vi "运维调试_五参数.vi"() -> ()   [LabVIEW 2016, in "斯坦道仪器.lvlib"]
uses:
  <vilib>/Utility/miscctls.llb/LVPointTypeDef.ctl
  PLC/PLC.lvlib
panel:
  in  "打开串口":bool
  in  "释放串口":bool
  in  "手动通电":bool
  out "多参数横条运行状态":T1(xcontrol)
  in  "数据区":i32(listbox)
  in  "探头选择":u16(ring)=9 items=["氨氮"=3, "水温"=9, "pH值"=10, "溶解氧"=11, "电导率"=12, "浊度"=13, "叶绿素a"=14, "藻密度"=15, "蓝绿藻"=16, "氧化还原电位"=17, "溶解氧%"=18, "盐度"=19]
  in  "测量数据区读取":bool
  in  "测量数据区":i32(listbox)
  in  "状态告警区读取":bool
  in  "状态告警区":i32(listbox)
  in  "自动校准":bool
  in  "读取KB":bool
  in  "写入KB":bool
  out "B":dbl caption="校准值B:"
  out "K":dbl caption="校准值K:"
  in  "校准区探头选择":u16(ring)=9 items=["氨氮"=3, "水温"=9, "pH值"=10, "电导率"=12, "浊度"=13, "叶绿素a"=14, "藻密度"=15, "蓝绿藻"=16, "氧化还原电位"=17, "溶解氧%"=18, "盐度"=19]
  in  "停止测量(单探)":bool
  in  "启动测量(单探)":bool
  in  "控制命令区探头选择":u16(ring)=9 items=["氨氮"=3, "水温"=9, "pH值"=10, "溶解氧"=11, "电导率"=12, "浊度"=13, "叶绿素a"=14, "藻密度"=15, "蓝绿藻"=16, "氧化还原电位"=17, "溶解氧%"=18, "盐度"=19]
  in  "同步时间":bool
  in  "初始化(清洗)":bool
  in  "停止测量(全部)":bool
  in  "启动测量(全部)":bool
  in  "关键参数区读取":bool
  in  "关键参数区":i32(listbox)
  in  "传感器参数读取":bool
  in  "传感器区":i32(listbox)
  in  "返回":bool
  in  "设置":bool
  out "运行状态":string
  out "开机状态":bool
  in  "停止":bool
  in  "手动启动":bool
  out "集成报警信息":string
  # "控制命令区"
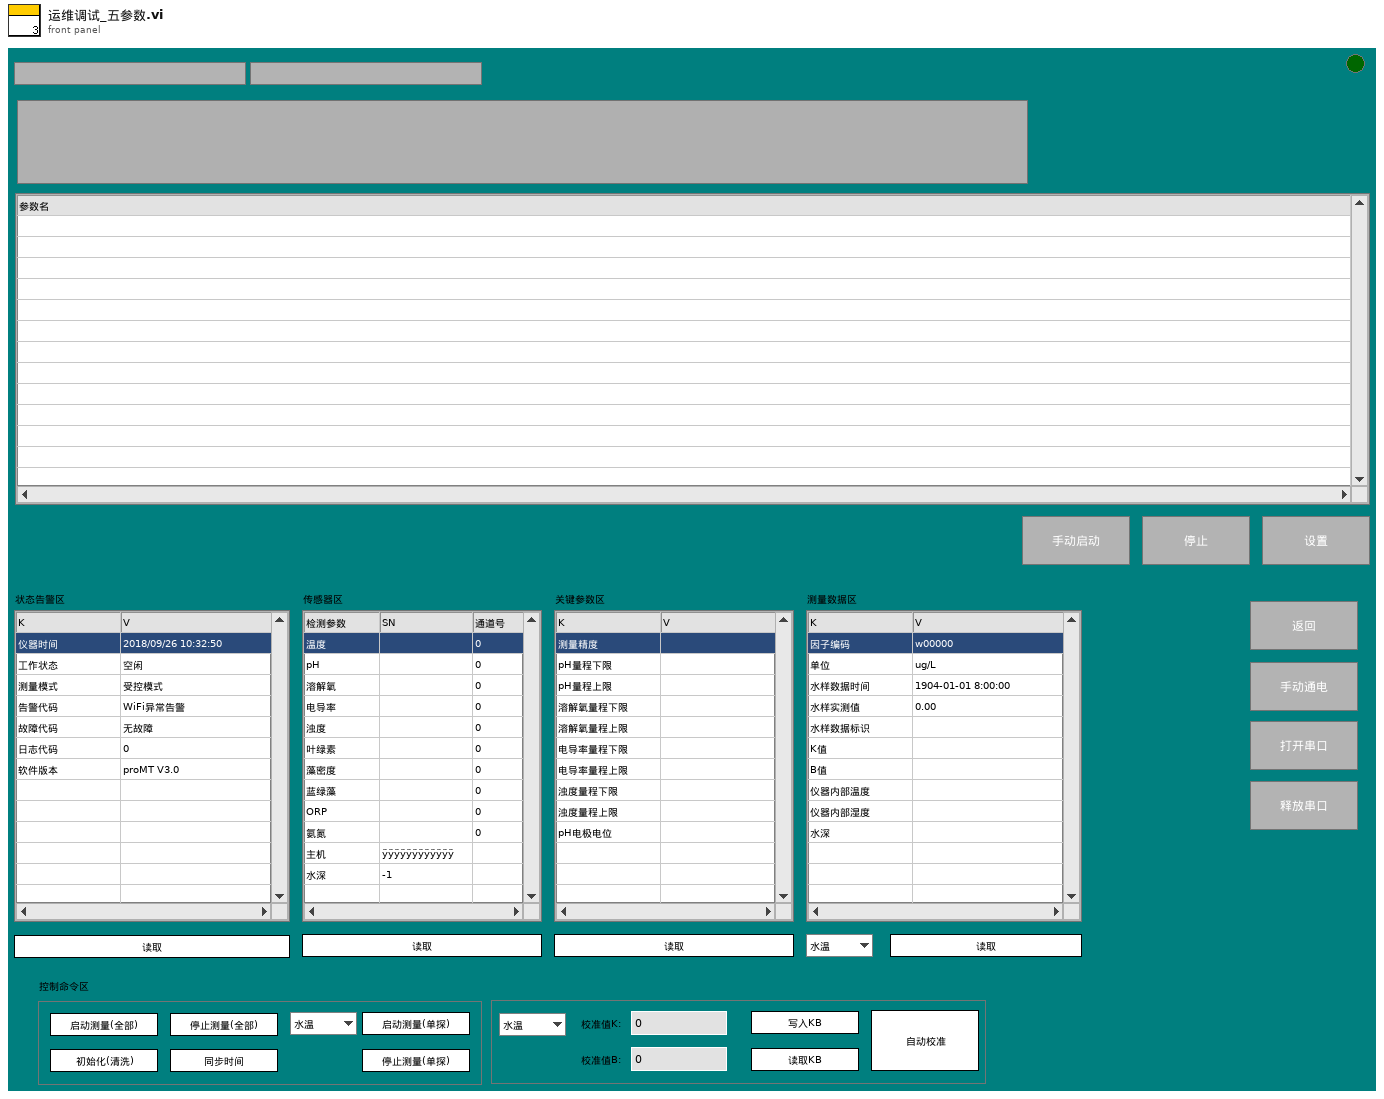
[diagram p1: front panel]
types:
  T1 = cluster{"系统时间":timestamp, "工作状态":u16, "测量模式":u16, "告警代码":enum16{"无告警", "缺试剂告警", "缺水样告警", "缺蒸馏水告警", "缺标液告警", "仪表漏液告警", "标定异常告警", "超量程告警", "加热异常", "低试剂预警", "超上限告警", "超下限告警", "仪表内部其他异常", "滴定异常告警", "电极异常告警", "量程切换告警", "参数设置告警", "PH电极电位异常", "电导率电极异常", "浊度光度异常", "溶解氧电极异常", "溶解氧光强异常", "温度异常告警", "PH异常告警", "溶解氧异常告警", "电导率异常告警", "浊度异常告警", "叶绿素异常告警", "藻密度异常告警", "蓝绿藻异常告警", "ORP异常告警", "氨氮异常告警", "清洁刷异常告警", "SD卡异常告警", "蓝牙异常告警", "Wifi异常告警", "流程异常告警"}, "故障代码":enum16{"无故障", "电机故障", "温度故障", "通讯故障", "滴定故障"}, "日志代码":u16, "软件版本":string}
  T2 = typedef "LVPointTypeDef.ctl" = cluster{"Horizontal":i16, "Vertical":i16}
  T3 = cluster{"时间标识":timestamp, "设备":string, "日志信息":string}
  T4 = enum16{"无告警", "缺试剂告警", "缺水样告警", "缺蒸馏水告警", "缺标液告警", "仪表漏液告警", "标定异常告警", "超量程告警", "加热异常", "低试剂预警", "超上限告警", "超下限告警", "仪表内部其他异常", "滴定异常告警", "电极异常告警", "量程切换告警", "参数设置告警", "PH电极电位异常", "电导率电极异常", "浊度光度异常", "溶解氧电极异常", "溶解氧光强异常", "温度异常告警", "PH异常告警", "溶解氧异常告警", "电导率异常告警", "浊度异常告警", "叶绿素异常告警", "藻密度异常告警", "蓝绿藻异常告警", "ORP异常告警", "氨氮异常告警", "清洁刷异常告警", "SD卡异常告警", "蓝牙异常告警", "Wifi异常告警", "流程异常告警"}
  T5 = cluster{"WORD[0]":u16, "WORD[1]":u16, "WORD[2]":u16, "WORD[3]":u16, "WORD[4]":u16, "WORD[5]":u16, "WORD[6]":u16, "WORD[7]":u16, "WORD[8]":u16, "WORD[9]":u16}
  T6 = cluster{"因子编码":string, "单位":string, "标样参考值":sgl, "水样数据时间":timestamp, "水样实测值":sgl, "水样数据标识":string, "K":sgl, "B":sgl, "T":sgl, "H":sgl, "水深":sgl}
  T7 = enum8{"Enabled", "Disabled", "Disabled and Grayed Out"}
  T8 = cluster{"测量模式":enum16{"待机", "水样测试", "标样核查", "零点核查", "跨度核查", "空白测试", "平行样测试", "加标回收", "空白校准", "标样校准", "初始化（清洗）"}, "数据标记表":string, "测量时间":dbl}
  T9 = cluster{"starting address":u16, "holding register value":u16}
  T10 = enum16{"idle", "init", "读状态", "读参数", "多个写入", "单个写入", "线圈写入"}
  T11 = enum32{"Bad", "Idle", "Run top level", "Running"}
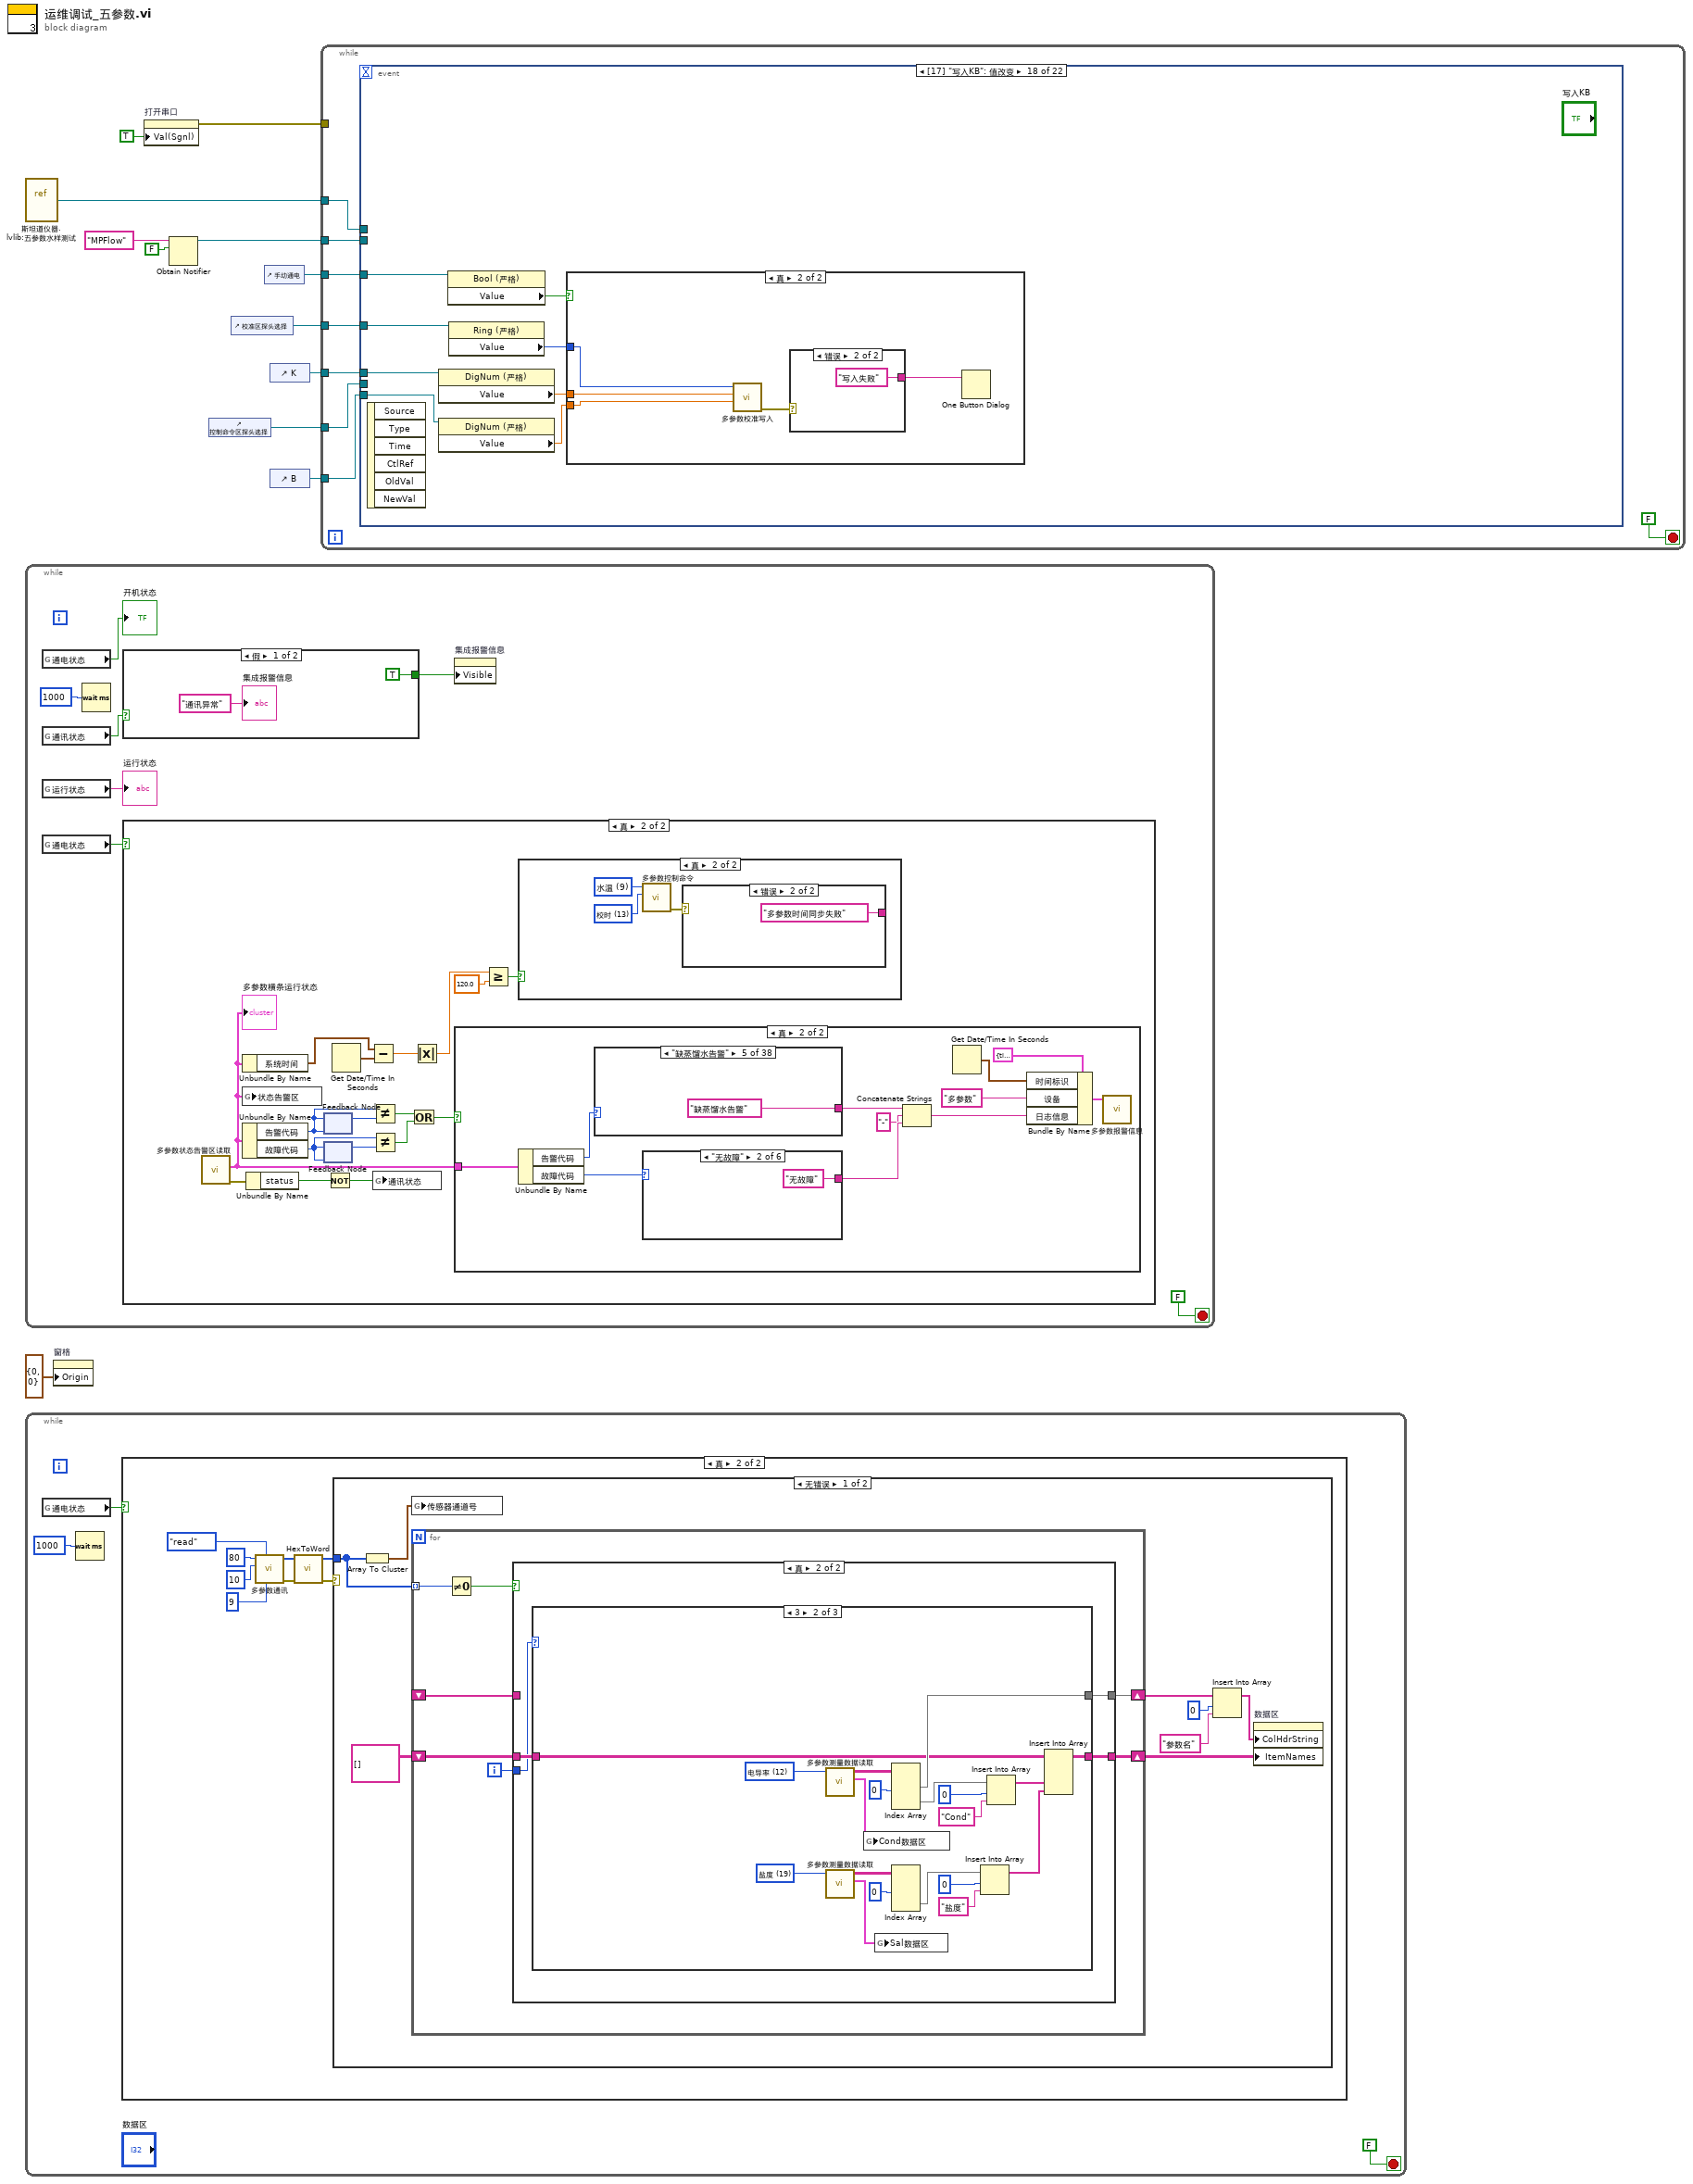
[diagram p0: block diagram]
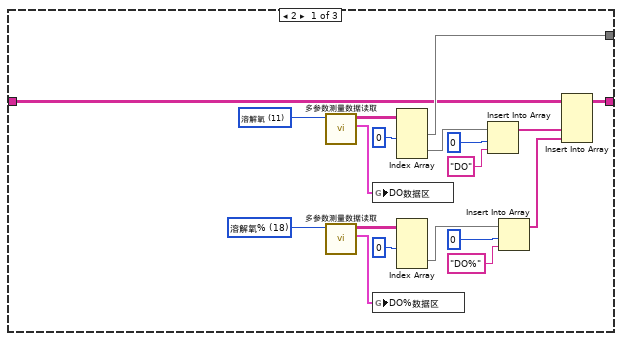
[diagram p4: hidden frame]
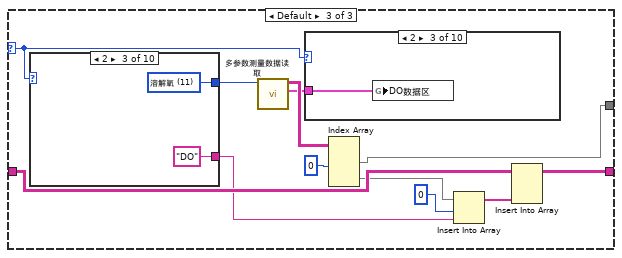
[diagram p5: hidden frame]
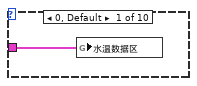
[diagram p6: hidden frame]
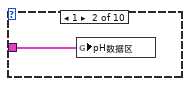
[diagram p7: hidden frame]
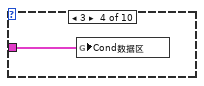
[diagram p8: hidden frame]
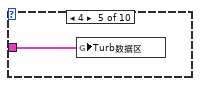
[diagram p9: hidden frame]
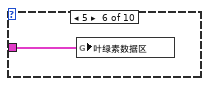
[diagram p10: hidden frame]
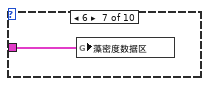
[diagram p11: hidden frame]
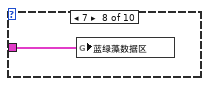
[diagram p12: hidden frame]
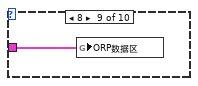
[diagram p13: hidden frame]
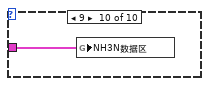
[diagram p14: hidden frame]
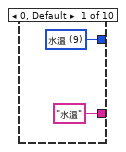
[diagram p15: hidden frame]
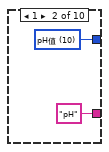
[diagram p16: hidden frame]
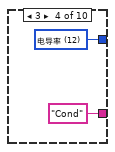
[diagram p17: hidden frame]
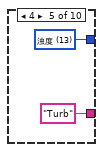
[diagram p18: hidden frame]
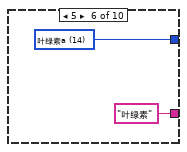
[diagram p19: hidden frame]
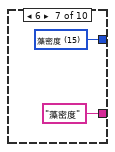
[diagram p20: hidden frame]
diagram:
  n1 = vi-ref "斯坦道仪器.lvlib:五参数水样测试.vi"() -> (w9:refnum<vi>)
  n2 = while {
    stop <- FALSE stop-if-true
    n3 = global read "多参数全局变量.vi" "通电状态"() -> (→"开机状态":bool)
    n4 = global read "多参数全局变量.vi" "通讯状态"() -> (w17:bool)
    n5 = global read "多参数全局变量.vi" "运行状态"() -> (→"运行状态":string)
    n6 = global read "多参数全局变量.vi" "通电状态"() -> (w13:bool)
    n7 = Wait (ms)(milliseconds to wait=u32 1000 ("等待时间（毫秒）")) -> ()  [unwired: 1 out]
    n8 = case shown="假" w17 {
      tunnel: [TRUE ("可见") _] -> w16
      frame False {
        "集成报警信息" <- "通讯异常" ("集成报警信息")
      }
      frame True {
      }
    }
    n9 = case shown="真" w13 {
      frame False {
      }
      frame True {
        n10 = call "多参数状态告警区读取.vi"() -> ("error out"=w29:errorcluster, "状态告警块"=w26:T1)  [unwired: 9 in, 1 out]
        "多参数横条运行状态" <- w26
        n11 = Unbundle By Name(w26) -> ("系统时间"=w25:timestamp)
        n12 = global write "多参数全局变量.vi" "状态告警区"(w26) -> ()
        n13 = Unbundle By Name(w26) -> ("告警代码"=w35:T4, "故障代码"=w33:enum16{"无故障", "电机故障", "温度故障", "通讯故障", "滴定故障"})
        n14 = Unbundle By Name(w29) -> ("status"=w28:bool)
        n15 = feedback #1(w35) -> (w36:T4)
        n16 = feedback-in #1(w35) -> ()
        n17 = feedback #2(w33) -> (w34:enum16{"无故障", "电机故障", "温度故障", "通讯故障", "滴定故障"})
        n18 = feedback-in #2(w33) -> ()
        n19 = Not(x=w28) -> (.not. x?=w27:bool)
        n20 = Get Date/Time In Seconds() -> (seconds since 1Jan1904=w24:timestamp)
        n21 = Subtract(x=w25, y=w24) -> (x-y=w23:dbl)
        n22 = Not Equal?(x=w35, y=w36) -> (x != y?=w31:bool)
        n23 = Not Equal?(x=w33, y=w34) -> (x != y?=w32:bool)
        n24 = global write "多参数全局变量.vi" "通讯状态"(w27) -> ()
        n25 = Or(x=w31, y=w32) -> (x .or. y?=w30:bool)
        n26 = Absolute Value(x=w23) -> (abs(x)=w22:dbl)
        n27 = case shown="真" w30 {
          tunnel: w26 -> [_ w52]
          frame False {
          }
          frame True {
            n28 = Unbundle By Name(w52) -> ("告警代码"=w51:T4, "故障代码"=w50:enum16{"无故障", "电机故障", "温度故障", "通讯故障", "滴定故障"})
            n29 = case shown="\"缺蒸馏水告警\"" w51 {
              selector: w51 -> [w63 _ _ _ _ _ _ _ _ _ _ _ _ _ _ _ _ _ _ _ _ _ _ _ _ _ _ _ _ _ _ _ _ _ _ _ _ _]
              tunnel: [w62 "无告警" "缺试剂告警" "缺水样告警" "缺蒸馏水告警" "缺标液告警" "仪表漏液告警" "标定异常告警" "超量程告警" "加热异常" "低试剂预警" "超上限告警" "超下限告警" "仪表内部其他异常" "滴定异常告警" "电极异常告警" "量程切换告警" "参数设置告警" "PH电极电位异常" "电导率电极异常" "浊度光度异常" "溶解氧电极异常" "溶解氧光强异常" "温度异常告警" "PH异常告警" "溶解氧异常告警" "电导率异常告警" "浊度异常告警" "叶绿素异常告警" "藻密度异常告警" "蓝绿藻异常告警" "ORP异常告警" "氨氮异常告警" "清洁刷异常告警" "SD卡异常告警" "蓝牙异常告警" "WiFi异常告警" "流程异常告警"] -> w49
              frame Default {
                n30 = Format Into String(format string="%d" ("格式字符串"), initial string="未知" ("工作状态"), w63) -> (resulting string=w62:string)  [unwired: 1 in, 1 out]
              }
              frame "无告警" {
              }
              frame "缺试剂告警" {
              }
              frame "缺水样告警" {
              }
              frame "缺蒸馏水告警" {
              }
              frame "缺标液告警" {
              }
              frame "仪表漏液告警" {
              }
              frame "标定异常告警" {
              }
              frame "超量程告警" {
              }
              frame "加热异常" {
              }
              frame "低试剂预警" {
              }
              frame "超上限告警" {
              }
              frame "超下限告警" {
              }
              frame "仪表内部其他异常" {
              }
              frame "滴定异常告警" {
              }
              frame "电极异常告警" {
              }
              frame "量程切换告警" {
              }
              frame "参数设置告警" {
              }
              frame "PH电极电位异常" {
              }
              frame "电导率电极异常" {
              }
              frame "浊度光度异常" {
              }
              frame "溶解氧电极异常" {
              }
              frame "溶解氧光强异常" {
              }
              frame "温度异常告警" {
              }
              frame "PH异常告警" {
              }
              frame "溶解氧异常告警" {
              }
              frame "电导率异常告警" {
              }
              frame "浊度异常告警" {
              }
              frame "叶绿素异常告警" {
              }
              frame "藻密度异常告警" {
              }
              frame "蓝绿藻异常告警" {
              }
              frame "ORP异常告警" {
              }
              frame "氨氮异常告警" {
              }
              frame "清洁刷异常告警" {
              }
              frame "SD卡异常告警" {
              }
              frame "蓝牙异常告警" {
              }
              frame "Wifi异常告警" {
              }
              frame "流程异常告警" {
              }
            }
            n31 = case shown="\"无故障\"" w50 {
              selector: w50 -> [w54 _ _ _ _ _]
              tunnel: [w53 "无故障" "电机故障" "温度故障" "通讯故障" "滴定故障"] -> w48
              frame Default {
                n32 = Format Into String(format string="%d" ("格式字符串"), initial string="未知" ("工作状态"), w54) -> (resulting string=w53:string)  [unwired: 1 in, 1 out]
              }
              frame "无故障" {
              }
              frame "电机故障" {
              }
              frame "温度故障" {
              }
              frame "通讯故障" {
              }
              frame "滴定故障" {
              }
            }
            n33 = Concatenate Strings(w49, "-" ("字符串"), w48) -> (w44:string)
            n34 = Get Date/Time In Seconds() -> (seconds since 1Jan1904=w43:timestamp)
            n35 = Bundle By Name(cluster=T3 {"时间标识"=timestamp(0 s since 1904-01-01), "设备"="", "日志信息"=""} ("data in"), "时间标识"=w43, "设备"="多参数", "日志信息"=w44) -> (w45:T3)
            n36 = call "多参数报警信息.vi"("data in"=w45) -> ()  [unwired: 10 in, 1 out]
          }
        }
        n37 = Greater Or Equal?(x=w22, y=120.0) -> (x >= y?=w21:bool)
        n38 = case shown="真" w21 {
          frame False {
          }
          frame True {
            w37 = u16 13 items=["启动测量（全部）"=1, "初始化（清洗）"=10, "停止测量（全部）"=11, "校时"=13, "启动测量（单个传感器）"=19, "停止测量（单个传感器）"=20] ("控制命令")
            w38 = u16 9 items=["氨氮"=3, "水温"=9, "pH值"=10, "溶解氧"=11, "电导率"=12, "浊度"=13, "叶绿素a"=14, "藻密度"=15, "蓝绿藻"=16, "氧化还原电位"=17, "溶解氧%"=18, "盐度"=19] ("站号")
            n39 = call "多参数控制命令.vi"("控制命令"=w37, "站号"=w38) -> ("error out"=w39:errorcluster)  [unwired: 9 in]
            n40 = case shown="错误" w39 {
              tunnel: ["多参数时间同步成功" ("消息") "多参数时间同步失败" ("消息")] -> _
              frame No Error {
              }
              frame Error {
              }
            }
          }
        }
      }
    }
    n41 = property on="集成报警信息" class="Str"("Visible"=w16) -> ()  [unwired: 2 in, 2 out]
  }
  n42 = while {
    stop <- FALSE stop-if-true
    n43 = global read "多参数全局变量.vi" "通电状态"() -> (w105:bool)
    n44 = Wait (ms)(milliseconds to wait=u32 1000 ("等待时间（毫秒）")) -> ()  [unwired: 1 out]
    n45 = case shown="真" w105 {
      frame False {
      }
      frame True {
        n46 = call "多参数通讯.vi"("Slave ID"=u8 9, "STEP"=enum16{"open", "read", "write", "close"}."read", "quantity"=u16 10, "starting address"=u16 80) -> ("error out"=w110:errorcluster, "Registers"=w111:u16[])  [unwired: 5 in, 1 out]
        n47 = call "HexToWord.vi"("数组"=w111) -> ("WORD"=w114:u16[])  [unwired: 10 in]
        n48 = case shown="无错误" w110 {
          tunnel: w114 -> [w115 _]
          frame No Error {
            n49 = Array To Cluster(array=w115) -> (cluster=w116:T5)
            n50 = global write "多参数全局变量.vi" "传感器通道号"(w116) -> ()
            n51 = for {
              tunnel: w115 -> [w128] mode=indexing
              shift-right: [w126] -> w120
              shift-left: _ -> [w125]
              shift-right: [w123] -> w121
              shift-left: string[][] [] ("子数组") -> [w124]
              i -> [w129]
              n52 = Not Equal To 0?(x=w128) -> (x != 0?=w127:bool)
              n53 = case shown="真" w127 {
                tunnel: w129 -> [_ w132]
                tunnel: [w131 w135] -> w126
                tunnel: w125 -> [w131 _]
                tunnel: w124 -> [w130 w134]
                tunnel: [w130 w133] -> w123
                frame False {
                }
                frame True {
                  n54 = case shown="3" w132 {
                    selector: w132 -> [_ _ w174]
                    tunnel: [w144 w163 w182] -> w135
                    tunnel: w134 -> [w140 w159 w181]
                    tunnel: [w143 w162 w180] -> w133
                    frame 2 {
                      w138 = u16 18 items=["氨氮"=3, "水温"=9, "pH值"=10, "溶解氧"=11, "电导率"=12, "浊度"=13, "叶绿素a"=14, "藻密度"=15, "蓝绿藻"=16, "氧化还原电位"=17, "溶解氧%"=18, "盐度"=19] ("探头选择")
                      w139 = u16 11 items=["氨氮"=3, "水温"=9, "pH值"=10, "溶解氧"=11, "电导率"=12, "浊度"=13, "叶绿素a"=14, "藻密度"=15, "蓝绿藻"=16, "氧化还原电位"=17, "溶解氧%"=18, "盐度"=19] ("探头选择")
                      n55 = call "多参数测量数据读取.vi"("探头选择"=w139) -> ("测量数据块"=w137:T6, "添加的数组"=w142:string[][])  [unwired: 8 in, 1 out]
                      n56 = call "多参数测量数据读取.vi"("探头选择"=w138) -> ("测量数据块"=w136:T6, "添加的数组"=w141:string[][])  [unwired: 8 in, 1 out]
                      n57 = global write "多参数全局变量.vi" "DO数据区"(w137) -> ()
                      n58 = global write "多参数全局变量.vi" "DO%数据区"(w136) -> ()
                      n59 = Index Array(array=w142, index (col) #1=0 ("禁用的索引 (列)")) -> (element #1=w144:string[], element #2=w153:string[])  [unwired: 3 in]
                      n60 = Index Array(array=w141, index (col) #1=0 ("禁用的索引 (列)")) -> (element #2=w149:string[])  [unwired: 3 in, 1 out]
                      n61 = Insert Into Array(array=w153, index=0 ("索引"), new element="DO") -> (w151:string[])
                      n62 = Insert Into Array(array=w149, index=0 ("索引"), new element="DO%") -> (w148:string[])
                      n63 = Insert Into Array(array=w140, new element #1=w151, new element #2=w148) -> (w143:string[][])  [unwired: 2 in]
                    }
                    frame 3 {
                      w157 = u16 19 items=["氨氮"=3, "水温"=9, "pH值"=10, "溶解氧"=11, "电导率"=12, "浊度"=13, "叶绿素a"=14, "藻密度"=15, "蓝绿藻"=16, "氧化还原电位"=17, "溶解氧%"=18, "盐度"=19] ("探头选择")
                      w158 = u16 12 items=["氨氮"=3, "水温"=9, "pH值"=10, "溶解氧"=11, "电导率"=12, "浊度"=13, "叶绿素a"=14, "藻密度"=15, "蓝绿藻"=16, "氧化还原电位"=17, "溶解氧%"=18, "盐度"=19] ("探头选择")
                      n64 = call "多参数测量数据读取.vi"("探头选择"=w158) -> ("测量数据块"=w156:T6, "添加的数组"=w161:string[][])  [unwired: 8 in, 1 out]
                      n65 = call "多参数测量数据读取.vi"("探头选择"=w157) -> ("测量数据块"=w155:T6, "添加的数组"=w160:string[][])  [unwired: 8 in, 1 out]
                      n66 = global write "多参数全局变量.vi" "Cond数据区"(w156) -> ()
                      n67 = global write "多参数全局变量.vi" "Sal数据区"(w155) -> ()
                      n68 = Index Array(array=w161, index (col) #1=0 ("禁用的索引 (列)")) -> (element #1=w163:string[], element #2=w172:string[])  [unwired: 3 in]
                      n69 = Index Array(array=w160, index (col) #1=0 ("禁用的索引 (列)")) -> (element #2=w168:string[])  [unwired: 3 in, 1 out]
                      n70 = Insert Into Array(array=w168, index=0 ("索引"), new element="盐度") -> (w167:string[])
                      n71 = Insert Into Array(array=w172, index=0 ("索引"), new element="Cond") -> (w170:string[])
                      n72 = Insert Into Array(array=w159, new element #1=w170, new element #2=w167) -> (w162:string[][])  [unwired: 2 in]
                    }
                    frame Default {
                      n73 = case shown="2" w174 {
                        tunnel: [w197 w199 w201 w203 w205 w207 w209 w211 w213 w215] -> w185
                        tunnel: ["水温" "pH" "DO" "Cond" "Turb" "叶绿素" "藻密度" "蓝绿藻" "ORP" "氨氮"] -> w178
                        frame 0, Default {
                          w197 = u16 9 items=["氨氮"=3, "水温"=9, "pH值"=10, "溶解氧"=11, "电导率"=12, "浊度"=13, "叶绿素a"=14, "藻密度"=15, "蓝绿藻"=16, "氧化还原电位"=17, "溶解氧%"=18, "盐度"=19] ("探头选择")
                        }
                        frame 1 {
                          w199 = u16 10 items=["氨氮"=3, "水温"=9, "pH值"=10, "溶解氧"=11, "电导率"=12, "浊度"=13, "叶绿素a"=14, "藻密度"=15, "蓝绿藻"=16, "氧化还原电位"=17, "溶解氧%"=18, "盐度"=19] ("探头选择")
                        }
                        frame 2 {
                          w201 = u16 11 items=["氨氮"=3, "水温"=9, "pH值"=10, "溶解氧"=11, "电导率"=12, "浊度"=13, "叶绿素a"=14, "藻密度"=15, "蓝绿藻"=16, "氧化还原电位"=17, "溶解氧%"=18, "盐度"=19] ("探头选择")
                        }
                        frame 3 {
                          w203 = u16 12 items=["氨氮"=3, "水温"=9, "pH值"=10, "溶解氧"=11, "电导率"=12, "浊度"=13, "叶绿素a"=14, "藻密度"=15, "蓝绿藻"=16, "氧化还原电位"=17, "溶解氧%"=18, "盐度"=19] ("探头选择")
                        }
                        frame 4 {
                          w205 = u16 13 items=["氨氮"=3, "水温"=9, "pH值"=10, "溶解氧"=11, "电导率"=12, "浊度"=13, "叶绿素a"=14, "藻密度"=15, "蓝绿藻"=16, "氧化还原电位"=17, "溶解氧%"=18, "盐度"=19] ("探头选择")
                        }
                        frame 5 {
                          w207 = u16 14 items=["氨氮"=3, "水温"=9, "pH值"=10, "溶解氧"=11, "电导率"=12, "浊度"=13, "叶绿素a"=14, "藻密度"=15, "蓝绿藻"=16, "氧化还原电位"=17, "溶解氧%"=18, "盐度"=19] ("探头选择")
                        }
                        frame 6 {
                          w209 = u16 15 items=["氨氮"=3, "水温"=9, "pH值"=10, "溶解氧"=11, "电导率"=12, "浊度"=13, "叶绿素a"=14, "藻密度"=15, "蓝绿藻"=16, "氧化还原电位"=17, "溶解氧%"=18, "盐度"=19] ("探头选择")
                        }
                        frame 7 {
                          w211 = u16 16 items=["氨氮"=3, "水温"=9, "pH值"=10, "溶解氧"=11, "电导率"=12, "浊度"=13, "叶绿素a"=14, "藻密度"=15, "蓝绿藻"=16, "氧化还原电位"=17, "溶解氧%"=18, "盐度"=19] ("探头选择")
                        }
                        frame 8 {
                          w213 = u16 17 items=["氨氮"=3, "水温"=9, "pH值"=10, "溶解氧"=11, "电导率"=12, "浊度"=13, "叶绿素a"=14, "藻密度"=15, "蓝绿藻"=16, "氧化还原电位"=17, "溶解氧%"=18, "盐度"=19] ("探头选择")
                        }
                        frame 9 {
                          w215 = u16 3 items=["氨氮"=3, "水温"=9, "pH值"=10, "溶解氧"=11, "电导率"=12, "浊度"=13, "叶绿素a"=14, "藻密度"=15, "蓝绿藻"=16, "氧化还原电位"=17, "溶解氧%"=18, "盐度"=19] ("探头选择")
                        }
                      }
                      n74 = call "多参数测量数据读取.vi"("探头选择"=w185) -> ("测量数据块"=w175:T6, "添加的数组"=w184:string[][])  [unwired: 8 in, 1 out]
                      n75 = case shown="2" w174 {
                        tunnel: w175 -> [w186 w187 w188 w189 w190 w191 w192 w193 w194 w195]
                        frame 0, Default {
                          n76 = global write "多参数全局变量.vi" "水温数据区"(w186) -> ()
                        }
                        frame 1 {
                          n77 = global write "多参数全局变量.vi" "pH数据区"(w187) -> ()
                        }
                        frame 2 {
                          n78 = global write "多参数全局变量.vi" "DO数据区"(w188) -> ()
                        }
                        frame 3 {
                          n79 = global write "多参数全局变量.vi" "Cond数据区"(w189) -> ()
                        }
                        frame 4 {
                          n80 = global write "多参数全局变量.vi" "Turb数据区"(w190) -> ()
                        }
                        frame 5 {
                          n81 = global write "多参数全局变量.vi" "叶绿素数据区"(w191) -> ()
                        }
                        frame 6 {
                          n82 = global write "多参数全局变量.vi" "藻密度数据区"(w192) -> ()
                        }
                        frame 7 {
                          n83 = global write "多参数全局变量.vi" "蓝绿藻数据区"(w193) -> ()
                        }
                        frame 8 {
                          n84 = global write "多参数全局变量.vi" "ORP数据区"(w194) -> ()
                        }
                        frame 9 {
                          n85 = global write "多参数全局变量.vi" "NH3N数据区"(w195) -> ()
                        }
                      }
                      n86 = Index Array(array=w184, index (col) #1=0 ("禁用的索引 (列)")) -> (element #1=w182:string[], element #2=w179:string[])  [unwired: 3 in]
                      n87 = Insert Into Array(array=w179, index=0 ("索引"), new element=w178) -> (w177:string[])
                      n88 = Insert Into Array(array=w181, new element=w177) -> (w180:string[][])  [unwired: 2 in]
                    }
                  }
                }
              }
            }
            n89 = Insert Into Array(array=w120, index=0 ("索引"), new element="参数名" ("新元素/子数组")) -> (w119:string[])
            n90 = property on="数据区" class="MCListbox (严格)"("ColHdrString"=w119, "ItemNames"=w121) -> ()  [unwired: 2 in, 2 out]
          }
          frame Error {
          }
        }
      }
    }
  }
  n91 = property on="窗格" class="Pane"("Origin"=T2 {"Horizontal"=0, "Vertical"=0} ("原点")) -> ()  [unwired: 2 in, 2 out]
  n92 = property on="打开串口" class="Bool (严格)"("Val(Sgnl)"=TRUE ("值(信号)")) -> (error out=w1:errorcluster)  [unwired: 2 in, 1 out]
  n93 = Obtain Notifier(name (unnamed)="MPFlow" ("名称（未命名）"), notification data type=FALSE) -> (notifier out=w8:refnum<notifier>)  [unwired: 2 in, 2 out]
  n94 = control-ref of="控制命令区探头选择"() -> (w7:refnum<vi>)
  n95 = control-ref of="校准区探头选择"() -> (w4:refnum<vi>)
  n96 = control-ref of="手动通电"() -> (w3:refnum<vi>)
  n97 = control-ref of="K"() -> (w6:refnum<vi>)
  n98 = control-ref of="B"() -> (w5:refnum<vi>)
  n99 = while {
    tunnel: w9 -> [w222]
    tunnel: w8 -> [w221]
    tunnel: w7 -> [w220]
    tunnel: w6 -> [w219]
    tunnel: w5 -> [w218]
    tunnel: w4 -> [w217]
    tunnel: w3 -> [w216]
    tunnel: w1 -> [_]
    stop <- FALSE stop-if-true
    n100 = event shown="[17] \"写入KB\": 值改变" {
      selector: _ -> [_ _ _ _ _ _ _ _ _ _ _ _ _ _ _ _ _ _ _ _ _ _]
      dyn-events: _ -> [_ _ _ _ _ _ _ _ _ _ _ _ _ _ _ _ _ _ _ _ _ _]
      timeout: _ -> [_ _ _ _ _ _ _ _ _ _ _ _ _ _ _ _ _ _ _ _ _ _]
      tunnel: w222 -> [_ _ _ w238 _ _ _ _ _ _ _ _ _ _ _ _ _ _ _ _ _ _]
      tunnel: w221 -> [_ _ _ _ w260 _ _ _ _ _ _ _ _ _ _ _ _ _ _ _ _ _]
      tunnel: w220 -> [_ _ _ _ _ _ _ _ _ _ _ _ _ _ _ w324 w338 _ _ _ _ _]
      tunnel: w219 -> [_ _ _ _ _ _ _ _ _ _ _ _ _ _ _ _ _ w349 _ _ _ _]
      tunnel: w218 -> [_ _ _ _ _ _ _ _ _ _ _ _ _ _ _ _ _ w351 _ _ _ _]
      tunnel: w217 -> [_ _ _ _ _ _ _ _ _ _ _ _ _ _ _ _ _ w353 _ w369 _ _]
      tunnel: w216 -> [_ _ _ _ _ _ _ w268 w273 w278 w284 w289 w298 w307 w316 w326 w336 w347 _ w367 w379 _]
      event Timeout {
        n101 = event-data() -> ()  [unwired: 1 in, 3 out]
      }
      event "释放串口": Value Change {
        n102 = event-data() -> ("NewVal"=w224:bool)  [unwired: 1 in, 5 out]
        n103 = case shown="真" w224 {
          frame False {
          }
          frame True {
            n104 = call "多参数通讯.vi"("STEP"=enum16{"open", "read", "write", "close"}."close") -> ("error out"=w225:errorcluster)  [unwired: 8 in, 2 out]
            n105 = case shown="无错误" w225 {
              frame No Error {
                n106 = property on="打开串口" class="Bool (严格)"("DisabledEnum"=T7."Enabled" ("禁用")) -> ()  [unwired: 2 in, 2 out]
              }
              frame Error {
              }
            }
          }
        }
      }
      event "打开串口": Value Change {
        n107 = event-data() -> ("NewVal"=w228:bool)  [unwired: 1 in, 5 out]
        n108 = case shown="真" w228 {
          frame False {
          }
          frame True {
            n109 = call "多参数通讯.vi"("STEP"=enum16{"open", "read", "write", "close"}."open") -> ("error out"=w229:errorcluster)  [unwired: 8 in, 2 out]
            n110 = case shown="错误" w229 {
              tunnel: [T7."Disabled and Grayed Out" ("禁用") T7."Enabled" ("禁用")] -> w231
              frame No Error {
              }
              frame Error {
                n111 = One Button Dialog(message="多参数串口打开失败" ("消息")) -> ()  [unwired: 1 in, 1 out]
              }
            }
            n112 = property on="打开串口" class="Bool (严格)"("DisabledEnum"=w231, "Value"=FALSE ("打开串口")) -> ()  [unwired: 2 in, 2 out]
          }
        }
      }
      event "手动启动": Value Change {
        n113 = event-data() -> ()  [unwired: 1 in, 6 out]
        n114 = call "多参数启动参数对话框.vi"() -> ("确认"=w237:bool, "测量时间"=w236:dbl)  [unwired: 10 in]
        n115 = case shown="真" w237 {
          tunnel: w238 -> [_ w240]
          tunnel: w236 -> [_ w239]
          frame False {
          }
          frame True {
            n116 = property class="VI"(reference=w240) -> ("Name"=w244:string, "Exec.State"=w242:T11)  [unwired: 1 in, 2 out]
            n117 = Open VI Reference(type specifier VI Refnum (for type only)=refnum<vi> refnum ("类型说明符VI引用句柄（仅用于类型）"), vi path=w244, options=128 ("选项")) -> (vi reference=w243:refnum<vi>)  [unwired: 3 in, 1 out]
            n118 = case shown="\"Idle\"" w242 {
              tunnel: w243 -> [w248 w255]
              tunnel: [w248 w254] -> w241
              tunnel: w239 -> [_ w249]
              frame "Bad", Default {
                n119 = One Button Dialog(message="仪器已经启动，无需重复启动" ("消息")) -> ()  [unwired: 1 in, 1 out]
              }
              frame "Idle" {
                n120 = global read "系统变量.vi" "运行模式"() -> (w251:enum16{"维护模式", "常规模式", "应急模式", "质控模式"})
                n121 = case shown="\"常规模式\", 默认" w251 {
                  tunnel: ["M" ("数据标记表") "hd" ("数据标记表")] -> w250
                  frame "维护模式" {
                  }
                  frame "常规模式", Default {
                  }
                }
                n122 = Bundle By Name(cluster=T8 {"测量模式"=enum."水样测试", "数据标记表"="", "测量时间"=0.0} ("启动参数"), "数据标记表"=w250, "测量时间"=w249) -> (w252:T8)
                n123 = call-by-ref "开始异步调用"(reference=w255, "启动参数"=w252) -> (reference out=w254:refnum<vi>)  [unwired: 12 in, 1 out]
              }
            }
            n124 = Close Reference(reference=w241) -> ()  [unwired: 1 in, 1 out]
          }
        }
      }
      event "停止": Value Change {
        n125 = event-data() -> ()  [unwired: 1 in, 6 out]
        n126 = Two Button Dialog(message="请再一次确认是否停止测量" ("消息")) -> (T button?=w258:bool)  [unwired: 2 in]
        n127 = case shown="真" w258 {
          tunnel: w260 -> [_ w263]
          frame False {
          }
          frame True {
            w261 = u16 11 items=["启动测量（全部）"=1, "初始化（清洗）"=10, "停止测量（全部）"=11, "校时"=13, "启动测量（单个传感器）"=19, "停止测量（单个传感器）"=20] ("控制命令")
            w262 = u16 10 items=["氨氮"=3, "水温"=9, "pH值"=10, "溶解氧"=11, "电导率"=12, "浊度"=13, "叶绿素a"=14, "藻密度"=15, "蓝绿藻"=16, "氧化还原电位"=17, "溶解氧%"=18, "盐度"=19] ("站号")
            n128 = Send Notification(notification=TRUE ("通知"), notifier=w263) -> ()  [unwired: 1 in, 2 out]
            n129 = call "多参数控制命令.vi"("控制命令"=w261, "站号"=w262) -> ()  [unwired: 9 in, 1 out]
          }
        }
      }
      event "设置": Value Change {
        n130 = event-data() -> ()  [unwired: 1 in, 6 out]
        n131 = property on="窗格" class="Pane"("Origin"=T2 {"Horizontal"=0, "Vertical"=528} ("原点")) -> ()  [unwired: 2 in, 2 out]
      }
      event "返回": Value Change {
        n132 = event-data() -> ()  [unwired: 1 in, 6 out]
        n133 = property on="窗格" class="Pane"("Origin"=T2 {"Horizontal"=0, "Vertical"=0} ("原点")) -> ()  [unwired: 2 in, 2 out]
      }
      event "传感器参数读取": Value Change {
        n134 = event-data() -> ()  [unwired: 1 in, 6 out]
        n135 = property class="Bool (严格)"(reference=w268) -> ("Value"=w267:bool)  [unwired: 1 in, 2 out]
        n136 = case shown="真" w267 {
          frame False {
            n137 = One Button Dialog(message="启动失败，请先通电" ("消息")) -> ()  [unwired: 1 in, 1 out]
          }
          frame True {
            n138 = call "多参数传感器参数读取.vi"() -> ("error out"=w270:errorcluster, "添加的数组"=w271:string[][])  [unwired: 10 in]
            n139 = call <vilib>:"General Error Handler.vi"("error in (no error)"=w270) -> ()  [unwired: 10 in, 5 out]
            n140 = property on="传感器区" class="MCListbox (严格)"("ItemNames"=w271) -> ()  [unwired: 2 in, 2 out]
          }
        }
      }
      event "关键参数区读取": Value Change {
        n141 = event-data() -> ()  [unwired: 1 in, 6 out]
        n142 = property class="Bool (严格)"(reference=w273) -> ("Value"=w272:bool)  [unwired: 1 in, 2 out]
        n143 = case shown="假" w272 {
          frame False {
            n144 = One Button Dialog(message="启动失败，请先通电" ("消息")) -> ()  [unwired: 1 in, 1 out]
          }
          frame True {
            n145 = call "多参数关键参数读取.vi"() -> ("error out"=w275:errorcluster, "添加的数组"=w276:string[][])  [unwired: 10 in]
            n146 = call <vilib>:"General Error Handler.vi"("error in (no error)"=w275) -> ()  [unwired: 10 in, 5 out]
            n147 = property on="关键参数区" class="MCListbox (严格)"("ItemNames"=w276) -> ()  [unwired: 2 in, 2 out]
          }
        }
      }
      event "测量数据区读取": Value Change {
        n148 = event-data() -> ()  [unwired: 1 in, 6 out]
        n149 = property class="Bool (严格)"(reference=w278) -> ("Value"=w277:bool)  [unwired: 1 in, 2 out]
        n150 = case shown="假" w277 {
          frame False {
            n151 = One Button Dialog(message="启动失败，请先通电" ("消息")) -> ()  [unwired: 1 in, 1 out]
          }
          frame True {
            n152 = call "多参数测量数据读取.vi"("探头选择"="探头选择") -> ("error out"=w281:errorcluster, "添加的数组"=w282:string[][])  [unwired: 8 in, 1 out]
            n153 = call <vilib>:"General Error Handler.vi"("error in (no error)"=w281) -> ()  [unwired: 10 in, 5 out]
            n154 = property on="测量数据区" class="MCListbox (严格)"("ItemNames"=w282) -> ()  [unwired: 2 in, 2 out]
          }
        }
      }
      event "状态告警区读取": Value Change {
        n155 = event-data() -> ()  [unwired: 1 in, 6 out]
        n156 = property class="Bool (严格)"(reference=w284) -> ("Value"=w283:bool)  [unwired: 1 in, 2 out]
        n157 = case shown="真" w283 {
          frame False {
            n158 = One Button Dialog(message="启动失败，请先通电" ("消息")) -> ()  [unwired: 1 in, 1 out]
          }
          frame True {
            n159 = call "多参数状态告警区读取.vi"() -> ("error out"=w286:errorcluster, "添加的数组"=w287:string[][])  [unwired: 9 in, 1 out]
            n160 = call <vilib>:"General Error Handler.vi"("error in (no error)"=w286) -> ()  [unwired: 10 in, 5 out]
            n161 = property on="状态告警区" class="MCListbox (严格)"("ItemNames"=w287) -> ()  [unwired: 2 in, 2 out]
          }
        }
      }
      event "同步时间": Value Change {
        n162 = event-data() -> ()  [unwired: 1 in, 6 out]
        n163 = property class="Bool (严格)"(reference=w289) -> ("Value"=w288:bool)  [unwired: 1 in, 2 out]
        n164 = case shown="假" w288 {
          frame False {
            n165 = One Button Dialog(message="启动失败，请先通电" ("消息")) -> ()  [unwired: 1 in, 1 out]
          }
          frame True {
            w291 = u16 13 items=["启动测量（全部）"=1, "初始化（清洗）"=10, "停止测量（全部）"=11, "校时"=13, "启动测量（单个传感器）"=19, "停止测量（单个传感器）"=20] ("控制命令")
            w292 = u16 9 items=["氨氮"=3, "水温"=9, "pH值"=10, "溶解氧"=11, "电导率"=12, "浊度"=13, "叶绿素a"=14, "藻密度"=15, "蓝绿藻"=16, "氧化还原电位"=17, "溶解氧%"=18, "盐度"=19] ("站号")
            n166 = call "多参数控制命令.vi"("控制命令"=w291, "站号"=w292) -> ("error out"=w294:errorcluster)  [unwired: 9 in]
            n167 = case shown="错误" w294 {
              tunnel: ["时间同步成功" ("消息") "时间同步失败" ("消息")] -> w293
              frame No Error {
              }
              frame Error {
              }
            }
            n168 = One Button Dialog(message=w293) -> ()  [unwired: 1 in, 1 out]
          }
        }
      }
      event "启动测量(全部)": Value Change {
        n169 = event-data() -> ()  [unwired: 1 in, 6 out]
        n170 = property class="Bool (严格)"(reference=w298) -> ("Value"=w297:bool)  [unwired: 1 in, 2 out]
        n171 = case shown="假" w297 {
          frame False {
            n172 = One Button Dialog(message="启动失败，请先通电" ("消息")) -> ()  [unwired: 1 in, 1 out]
          }
          frame True {
            w300 = u16 1 items=["启动测量（全部）"=1, "初始化（清洗）"=10, "停止测量（全部）"=11, "校时"=13, "启动测量（单个传感器）"=19, "停止测量（单个传感器）"=20] ("控制命令")
            w301 = u16 9 items=["氨氮"=3, "水温"=9, "pH值"=10, "溶解氧"=11, "电导率"=12, "浊度"=13, "叶绿素a"=14, "藻密度"=15, "蓝绿藻"=16, "氧化还原电位"=17, "溶解氧%"=18, "盐度"=19] ("站号")
            n173 = call "多参数控制命令.vi"("控制命令"=w300, "站号"=w301) -> ("error out"=w303:errorcluster)  [unwired: 9 in]
            n174 = case shown="无错误" w303 {
              tunnel: ["启动成功" ("消息") "启动失败" ("消息")] -> w302
              frame No Error {
              }
              frame Error {
              }
            }
            n175 = One Button Dialog(message=w302) -> ()  [unwired: 1 in, 1 out]
          }
        }
      }
      event "停止测量(全部)": Value Change {
        n176 = event-data() -> ()  [unwired: 1 in, 6 out]
        n177 = property class="Bool (严格)"(reference=w307) -> ("Value"=w306:bool)  [unwired: 1 in, 2 out]
        n178 = case shown="真" w306 {
          frame False {
            n179 = One Button Dialog(message="启动失败，请先通电" ("消息")) -> ()  [unwired: 1 in, 1 out]
          }
          frame True {
            w311 = u16 11 items=["启动测量（全部）"=1, "初始化（清洗）"=10, "停止测量（全部）"=11, "校时"=13, "启动测量（单个传感器）"=19, "停止测量（单个传感器）"=20] ("控制命令")
            w312 = u16 9 items=["氨氮"=3, "水温"=9, "pH值"=10, "溶解氧"=11, "电导率"=12, "浊度"=13, "叶绿素a"=14, "藻密度"=15, "蓝绿藻"=16, "氧化还原电位"=17, "溶解氧%"=18, "盐度"=19] ("站号")
            n180 = call "多参数控制命令.vi"("控制命令"=w311, "站号"=w312) -> ("error out"=w310:errorcluster)  [unwired: 9 in]
            n181 = case shown="错误" w310 {
              tunnel: ["停止成功" ("消息") "停止失败" ("消息")] -> w309
              frame No Error {
              }
              frame Error {
              }
            }
            n182 = One Button Dialog(message=w309) -> ()  [unwired: 1 in, 1 out]
          }
        }
      }
      event "初始化(清洗)": Value Change {
        n183 = event-data() -> ()  [unwired: 1 in, 6 out]
        n184 = property class="Bool (严格)"(reference=w316) -> ("Value"=w315:bool)  [unwired: 1 in, 2 out]
        n185 = case shown="真" w315 {
          frame False {
            n186 = One Button Dialog(message="启动失败，请先通电" ("消息")) -> ()  [unwired: 1 in, 1 out]
          }
          frame True {
            w320 = u16 10 items=["启动测量（全部）"=1, "初始化（清洗）"=10, "停止测量（全部）"=11, "校时"=13, "启动测量（单个传感器）"=19, "停止测量（单个传感器）"=20] ("控制命令")
            w321 = u16 9 items=["氨氮"=3, "水温"=9, "pH值"=10, "溶解氧"=11, "电导率"=12, "浊度"=13, "叶绿素a"=14, "藻密度"=15, "蓝绿藻"=16, "氧化还原电位"=17, "溶解氧%"=18, "盐度"=19] ("站号")
            n187 = call "多参数控制命令.vi"("控制命令"=w320, "站号"=w321) -> ("error out"=w318:errorcluster)  [unwired: 9 in]
            n188 = case shown="错误" w318 {
              tunnel: ["初始化成功" ("消息") "初始化失败" ("消息")] -> w319
              frame No Error {
              }
              frame Error {
              }
            }
            n189 = One Button Dialog(message=w319) -> ()  [unwired: 1 in, 1 out]
          }
        }
      }
      event "启动测量(单探)": Value Change {
        n190 = event-data() -> ()  [unwired: 1 in, 6 out]
        n191 = property class="Bool (严格)"(reference=w326) -> ("Value"=w325:bool)  [unwired: 1 in, 2 out]
        n192 = property class="Ring (严格)"(reference=w324) -> ("Value"=w327:u16)  [unwired: 1 in, 2 out]
        n193 = case shown="真" w325 {
          tunnel: w327 -> [_ w329]
          frame False {
            n194 = One Button Dialog(message="启动失败，请先通电" ("消息")) -> ()  [unwired: 1 in, 1 out]
          }
          frame True {
            w330 = u16 19 items=["启动测量（全部）"=1, "初始化（清洗）"=10, "停止测量（全部）"=11, "校时"=13, "启动测量（单个传感器）"=19, "停止测量（单个传感器）"=20] ("控制命令")
            n195 = call "多参数控制命令.vi"("控制命令"=w330, "站号"=w329) -> ("error out"=w332:errorcluster)  [unwired: 9 in]
            n196 = case shown="无错误" w332 {
              tunnel: ["启动成功" ("消息") "启动失败" ("消息")] -> w331
              frame No Error {
              }
              frame Error {
              }
            }
            n197 = One Button Dialog(message=w331) -> ()  [unwired: 1 in, 1 out]
          }
        }
      }
      event "停止测量(单探)": Value Change {
        n198 = event-data() -> ()  [unwired: 1 in, 6 out]
        n199 = property class="Bool (严格)"(reference=w336) -> ("Value"=w335:bool)  [unwired: 1 in, 2 out]
        n200 = property class="Ring (严格)"(reference=w338) -> ("Value"=w337:u16)  [unwired: 1 in, 2 out]
        n201 = case shown="真" w335 {
          tunnel: w337 -> [_ w340]
          frame False {
            n202 = One Button Dialog(message="启动失败，请先通电" ("消息")) -> ()  [unwired: 1 in, 1 out]
          }
          frame True {
            w341 = u16 20 items=["启动测量（全部）"=1, "初始化（清洗）"=10, "停止测量（全部）"=11, "校时"=13, "启动测量（单个传感器）"=19, "停止测量（单个传感器）"=20] ("控制命令")
            n203 = call "多参数控制命令.vi"("控制命令"=w341, "站号"=w340) -> ("error out"=w343:errorcluster)  [unwired: 9 in]
            n204 = case shown="错误" w343 {
              tunnel: ["停止成功" ("消息") "停止失败" ("消息")] -> w342
              frame No Error {
              }
              frame Error {
              }
            }
            n205 = One Button Dialog(message=w342) -> ()  [unwired: 1 in, 1 out]
          }
        }
      }
      event "写入KB": Value Change {
        n206 = event-data() -> ()  [unwired: 1 in, 6 out]
        n207 = property class="DigNum (严格)"(reference=w349) -> ("Value"=w348:dbl)  [unwired: 1 in, 2 out]
        n208 = property class="DigNum (严格)"(reference=w351) -> ("Value"=w350:dbl)  [unwired: 1 in, 2 out]
        n209 = property class="Bool (严格)"(reference=w347) -> ("Value"=w346:bool)  [unwired: 1 in, 2 out]
        n210 = property class="Ring (严格)"(reference=w353) -> ("Value"=w352:u16)  [unwired: 1 in, 2 out]
        n211 = case shown="真" w346 {
          tunnel: w352 -> [_ w359]
          tunnel: w350 -> [_ w358]
          tunnel: w348 -> [_ w357]
          frame False {
            n212 = One Button Dialog(message="启动失败，请先通电" ("消息")) -> ()  [unwired: 1 in, 1 out]
          }
          frame True {
            n213 = call "多参数校准写入.vi"("B"=w358, "K"=w357, "站号"=w359) -> ("error out"=w355:errorcluster)  [unwired: 8 in]
            n214 = case shown="错误" w355 {
              tunnel: ["写入成功" ("消息") "写入失败" ("消息")] -> w356
              frame No Error {
              }
              frame Error {
              }
            }
            n215 = One Button Dialog(message=w356) -> ()  [unwired: 1 in, 1 out]
          }
        }
      }
      event "K", "B": Mouse Down {
        n216 = event-data() -> ("CtlRef"=w365:refnum<vi>)  [unwired: 1 in, 5 out]
        n217 = property class="DigNum (严格)"(reference=w365) -> (reference out=w364:refnum<vi>, "Value"=w363:dbl)  [unwired: 1 in, 1 out]
        n218 = call "数字键盘.vi"("OldNumber"=w363) -> ("NewNumber"=w362:sgl)
        n219 = property class="DigNum (严格)"(reference=w364, "Value"=w362) -> ()  [unwired: 1 in, 2 out]
      }
      event "读取KB": Value Change {
        n220 = event-data() -> ()  [unwired: 1 in, 6 out]
        n221 = property class="Bool (严格)"(reference=w367) -> ("Value"=w366:bool)  [unwired: 1 in, 2 out]
        n222 = property class="Ring (严格)"(reference=w369) -> ("Value"=w368:u16)  [unwired: 1 in, 2 out]
        n223 = case shown="真" w366 {
          tunnel: w368 -> [_ w373]
          frame False {
            n224 = One Button Dialog(message="启动失败，请先通电" ("消息")) -> ()  [unwired: 1 in, 1 out]
          }
          frame True {
            n225 = call "多参校准读取.vi"("站号"=w373) -> ("error out"=w371:errorcluster, "B"=→"B":dbl, "K"=→"K":dbl)  [unwired: 8 in]
            n226 = case shown="无错误" w371 {
              tunnel: ["读取成功" ("消息") "读取失败" ("消息")] -> w372
              frame No Error {
              }
              frame Error {
              }
            }
            n227 = One Button Dialog(message=w372) -> ()  [unwired: 1 in, 1 out]
          }
        }
      }
      event "自动校准": Value Change {
        n228 = event-data() -> ()  [unwired: 1 in, 6 out]
        n229 = property class="Bool (严格)"(reference=w379) -> ("Value"=w378:bool)  [unwired: 1 in, 2 out]
        n230 = case shown="真" w378 {
          frame False {
            n231 = One Button Dialog(message="启动失败，请先通电" ("消息")) -> ()  [unwired: 1 in, 1 out]
          }
          frame True {
            n232 = call "多参校准.vi"() -> ()  [unwired: 12 in]
          }
        }
      }
      event "手动通电": Value Change {
        n233 = event-data() -> ("NewVal"=w382:bool)  [unwired: 1 in, 5 out]
        n234 = Boolean To (0,1)(Boolean=w382) -> (0, 1=w381:i16)
        n235 = Bundle By Name(cluster=T9 {"starting address"=0, "holding register value"=0}, "starting address"=u16 302, "holding register value"=w381) -> (w384:T9)
        n236 = call "采配水通讯指令.vi"("数据"=w384, "命令"=T10."单个写入") -> ()  [unwired: 10 in]
      }
    }
  }
